vi "CSM - Module Status.vi"(8 "Error In":errorcluster caption="error in (no error)", 11 "CSM Name":string) -> (0 "error out":errorcluster, 1 "#Nodes":i32, 2 "Mode":T1=enum."Stand Alone", 3 "CSM Name (Dup)":string, 4 "#Elements In Queue":i32)   [LabVIEW 2017, in "Communicable State Machine.lvlib"]
doc: "### CSM - Module Status.vi\n\nGet the status of the CSM module, including: working mode, number of workers, and the number of pending messages in the message queue.\n\n> [!NOTE] CSM Working Modes\n> 1. Stand-alone: Independent working mode. If no module name is provided, a random ID will be generated to identify the module.\n> 2. CSM: Regular CSM module.\n> 3. Action Worker: Worker mode. Add \"#\" after the module name to mark this module as a worker, sharing the same message queue with other workers of the same name.\n> 4. Chain Node: Chain node. Add \"$\" after the module name to mark this module as a chain node. Messages on the same chain will be passed sequentially until a node processes the message.\n\n\n-- <b>Controls</b> --\n- <b>CSM Name</b>: CSM module name\n\n-- <b>Indicators</b> --\n- <b>Mode</b>: Returns the working mode of the module\n- <b>#As Worker</b>: Number of workers in worker mode for this module\n- <b>#msg to be processed</b>: Number of pending messages in the CSM message queue\n- <b>CSM Name(dup)</b>: Returns <b>CSM Name</b>"
uses:
  Communicable State Machine.lvlib
  _Support/Typedef/_CSM_MODE.ctl
  _Support/CSMQ/_CSMOFGVOPER.ctl
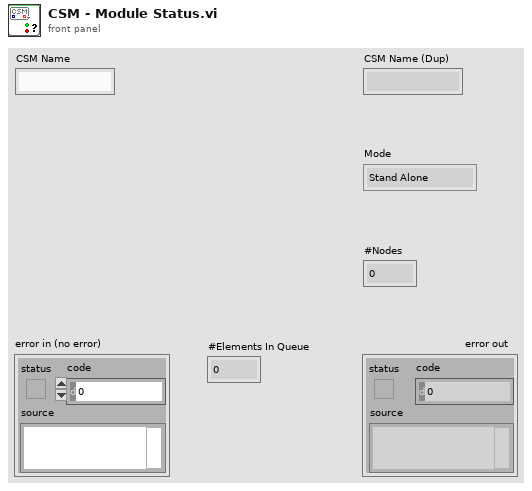
[diagram p1: front panel]
types:
  T1 = typedef "Communicable State Machine.lvlib/_CSM_MODE.ctl" = enum16{"Not Exist", "Stand Alone", "CSM", "Worker", "Worker Agent", "Chain Node", "Chain"}
  T2 = typedef "Communicable State Machine.lvlib/_CSMOFGVOPER.ctl" = enum16{"Create If not Exist", "Get By Name", "List", "Check If Name Exists", "Release", "Module Status", "Create Status Event Handler", "Destroy Status Event Handler", "Clear Invalid Objs"}
  T3 = typedef "Communicable State Machine.lvlib/_CSMObj.ctl" = cluster{"info":T4, "Refs":T5}
  T4 = typedef "Communicable State Machine.lvlib/_CSMObj-Info.ctl" = cluster{"Module Name":string, "Requested Name":string, "Group Name":string, "Mode":T1, "Allowed Messages":string[]}
  T5 = typedef "Communicable State Machine.lvlib/_CSMObj-Refs.ctl" = cluster{"WatchDogQ":refnum<queue>, "CSMDataDVR":refnum<data-value>, "Queue":T6, "GroupDataDVR":refnum<data-value>, "TagMap":refnum<data-value>, "ExitEvent":refnum<user-event>, "NewStateEvent":refnum<user-event>, "StatusChangeEvent":refnum<user-event>}
  T6 = typedef "Communicable State Machine.lvlib/Priority Queue.ctl" = cluster{"HPriorityQ":refnum<queue>, "LowPriorityQ":refnum<queue>}
  T7 = typedef "Communicable State Machine.lvlib/_CSMObj-ModeData.ctl" = cluster{"CSMDataDVR":refnum<data-value>[], "Messages of Chain Nodes":cluster{"Module Name":string, "Allowed Messages":string[]}[], "Chain Message Mapping Map":variant}
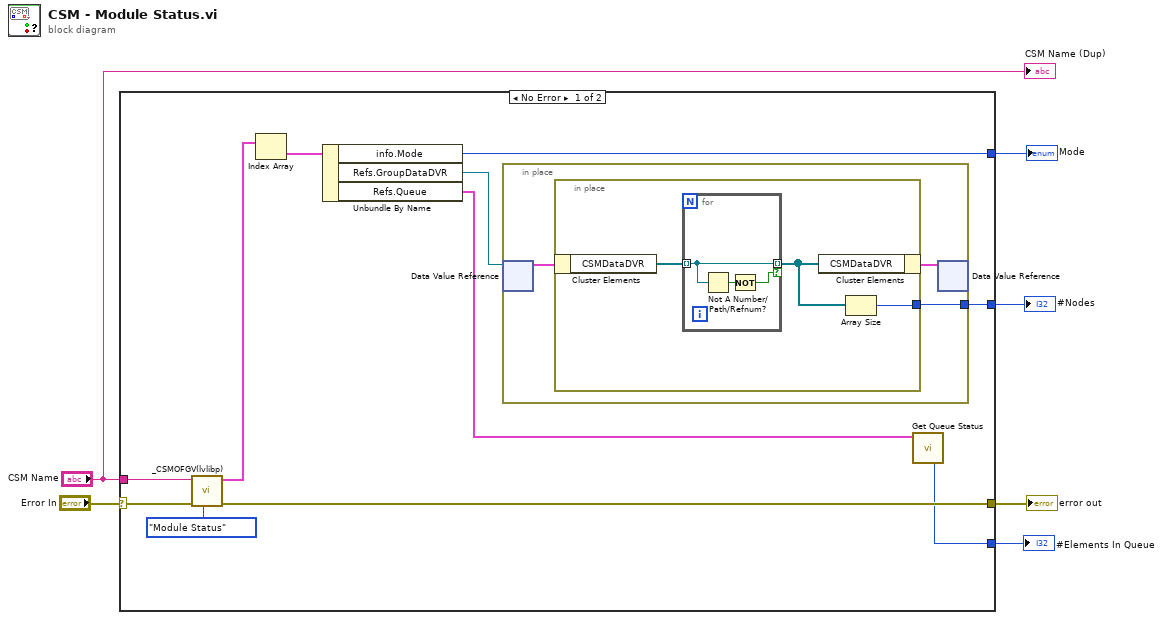
[diagram p0: block diagram]
diagram:
  n1 = case shown="No Error" "Error In" {
    selector: "Error In" -> [w17 w27]
    tunnel: [w16 w27] -> w5
    tunnel: [w12 _] -> w4
    tunnel: [w10 _] -> w3
    tunnel: "CSM Name" -> [w9 _]
    tunnel: [w7 _] -> w1
    frame No Error {
      n2 = call "_CSMOFGV(lvlibp).vi"("Operation"=_CSMOFGVOPER."Module Status", "Error In"=w17, "Name (\"\" to Use UUID) In"=w9) -> ("error out"=w16:errorcluster, "Array"=w14:T3[])  [unwired: 6 in, 1 out]
      n3 = Index Array(array=w14) -> (element=w13:T3)  [unwired: 1 in]
      n4 = Unbundle By Name(w13) -> ("info.Mode"=w12:T1, "Refs.GroupDataDVR"=w8:refnum<data-value>, "Refs.Queue"=w11:T6)
      n5 = in-place {
        in-place-border: [w18] -> w7
        n6 = in-place-dvr #1(w8) -> (w20:T7)  [unwired: 1 out]
        n7 = in-place {
          in-place-border: [w22] -> w18
          n8 = in-place-cluster #2(w20) -> ("CSMDataDVR"=w23:refnum<data-value>[])
          n9 = for {
            tunnel: [w26] -> w21 mode=indexing if=w24
            tunnel: w23 -> [w26] mode=indexing
            n10 = Not A Number/Path/Refnum?(number/path/refnum=w26) -> (NaN/Path/Refnum?=w25:bool)
            n11 = Not(x=w25) -> (.not. x?=w24:bool)
          }
          n12 = in-place-cluster #2("CSMDataDVR"=w21) -> (w19:T7)
          n13 = Array Size(array=w21) -> (size(s)=w22:i32)
        }
        n14 = in-place-dvr #1(w19) -> ()  [unwired: 2 out]
      }
      n15 = call "Get Queue Status.vi"("Priority Queue In"=w11) -> ("# Elements In Queue"=w10:i32)  [unwired: 6 in, 4 out]
    }
    frame Error {
    }
  }
  "error out" <- w5
  "Mode" <- w4
  "#Nodes" <- w1
  "#Elements In Queue" <- w3
  "CSM Name (Dup)" <- "CSM Name"
